vi "Counter - Continuous Output.vi"(9 "Frequency":dbl=10000.0 format="%.6f", 10 "Output Terminal":tag="/cDAQ1/Ctr0InternalOutput", 11 "Counter":tag="cDAQ1/_ctr0") -> (3 "Actual Frequency":dbl)   [LabVIEW 2014]
doc: "This example demonstrates how to continuously generate digital pulses using a counter output."
uses:
  <vilib>/DAQmx/create/channels.llb/DAQmx Create Channel (CO-Pulse Generation-Frequency).vi
  <vilib>/DAQmx/configure/timing.llb/DAQmx Timing (Implicit).vi
  <vilib>/DAQmx/configure/trigger.llb/DAQmx Start Trigger (Digital Edge).vi
  <resource>/objmgr/daqmx.rc
panel:
  out "Actual Duty Cycle":dbl
  in  "Duty Cycle":dbl=0.5 format="%.6f"
  in  "Trigger Type":T1(tab)
  in  "Edge":i32(ring)=10280 items=["Rising"=10280, "Falling"=10171]
  in  "Digital Trigger Source":tag
  in  "Pause When":i32(ring)=10192 items=["High"=10192, "Low"=10214]
  in  "Pause Trigger Source":tag
  in  "Stop":bool
  # "Channel Settings"
  # "Trigger Settings"
  # "To configure and use a trigger you must have the necessary tab selected above."
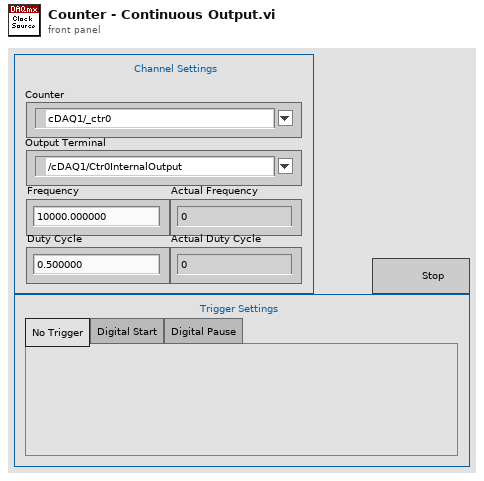
[diagram p1: front panel]
types:
  T1 = enum32{"No Trigger", "Digital Start", "Digital Pause"}
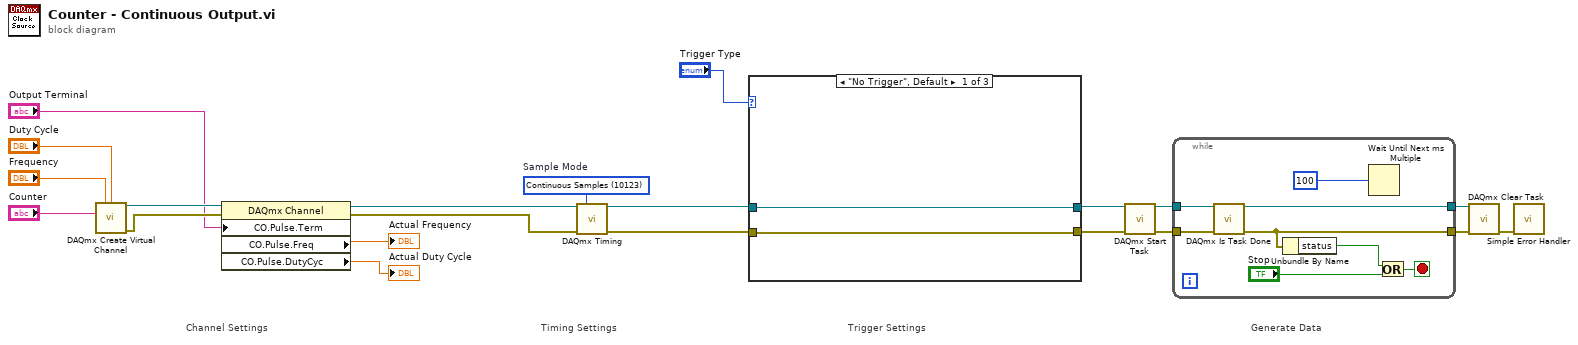
[diagram p0: block diagram]
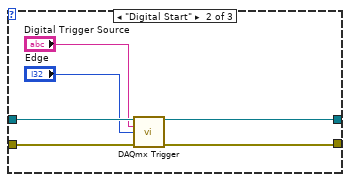
[diagram p2: hidden frame]
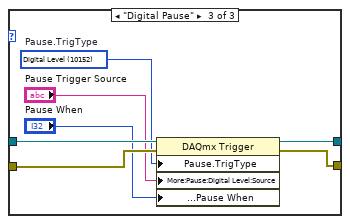
[diagram p3: hidden frame]
diagram:
  w21 = 10123 items=["Finite Samples"=10178, "Continuous Samples"=10123, "Hardware Timed Single Point"=12522]  # Sample Mode
  # "Generate Data"
  # "Trigger Settings"
  # "Timing Settings"
  # "Channel Settings"
  n1 = call-poly <vilib>:"DAQmx Create Virtual Channel.vi"("frequency"="Frequency", "duty cycle"="Duty Cycle", "counter"="Counter") -> ("task out"=w9:refnum<k21>, "error out"=w8:errorcluster)  [unwired: 11 in]
  n2 = property class="DAQmx Channel"(reference=w9, error in=w8, "CO.Pulse.Term"="Output Terminal") -> (reference out=w5:refnum<k21>, error out=w6:errorcluster, "CO.Pulse.Freq"=→"Actual Frequency":dbl, "CO.Pulse.DutyCyc"=→"Actual Duty Cycle":dbl)
  n3 = call-poly <vilib>:"DAQmx Timing.vi"("task/channels in"=w5, "sample mode"=w21, "error in"=w6) -> ("task out"=w13:refnum<k21>, "error out"=w12:errorcluster)  [unwired: 11 in]
  n4 = case shown="\"No Trigger\", Default" "Trigger Type" {
    tunnel: w13 -> [w23 w29 w36]
    tunnel: w12 -> [w22 w28 w33]
    tunnel: [w23 w27 w35] -> w10
    tunnel: [w22 w26 w34] -> w11
    frame "No Trigger", Default {
    }
    frame "Digital Start" {
      n5 = call-poly <vilib>:"DAQmx Trigger.vi"("task/channels in"=w29, "source"="Digital Trigger Source", "edge"="Edge", "error in"=w28) -> ("task out"=w27:refnum<k21>, "error out"=w26:errorcluster)  [unwired: 10 in]
    }
    frame "Digital Pause" {
      w32 = 10152 items=["Analog Level"=10101, "Analog Window"=10103, "Digital Level"=10152, "Digital Pattern"=10398, "None"=10230]  # Pause.TrigType
      n6 = property class="DAQmx Trigger"(reference=w36, error in=w33, "Pause.TrigType"=w32, "More:Pause:Digital Level:Source"="Pause Trigger Source", "More:Pause:Digital Level:Pause When"="Pause When") -> (reference out=w35:refnum<k21>, error out=w34:errorcluster)
    }
  }
  n7 = call <vilib>:"DAQmx Start Task.vi"("task/channels in"=w10, "error in"=w11) -> ("task out"=w20:refnum<k21>, "error out"=w19:errorcluster)  [unwired: 12 in]
  n8 = while {
    tunnel: w20 -> [w44]
    tunnel: w19 -> [w43]
    tunnel: [w41] -> w17
    tunnel: [w37] -> w18
    stop <- w42 stop-if-true
    n9 = call <vilib>:"DAQmx Is Task Done.vi"("task/channels in"=w44, "error in"=w43) -> ("task out"=w37:refnum<k21>, "error out"=w41:errorcluster)  [unwired: 11 in, 1 out]
    n10 = Unbundle By Name(w41) -> ("status"=w40:bool)
    n11 = Wait Until Next ms Multiple(millisecond multiple=u32 100) -> ()  [unwired: 1 out]
    n12 = Or(x=w40, y="Stop") -> (x .or. y?=w42:bool)
  }
  n13 = call <vilib>:"DAQmx Clear Task.vi"("task in"=w18, "error in"=w17) -> ("error out"=w16:errorcluster)  [unwired: 13 in]
  n14 = call <vilib>:"Simple Error Handler.vi"("error in (no error)"=w16) -> ()  [unwired: 4 in, 5 out]
